vi "Rotator.vi"() -> ()   [LabVIEW 2016]
uses:
  Libraries/Rotator/PerformaxLV_v102.llb/utility_actions.ctl
  Libraries/Rotator/PerformaxLV_v102.llb/commands.ctl
panel:
  in  "stop":bool
  in  "Tab Control":enum32{"Basic controls", "Advanced"}(tab)=enum."Advanced"
  out "In range":bool=TRUE
  out "Status":bool=TRUE
  in  "GO Button":bool
  in  "New position":dbl
  out "Current position":dbl
  in  "Min  angle":dbl=-5.1
  in  "Max angle":dbl=95.1
  in  "Steps per degree":dbl=-780.0
  in  "Redefine Button":bool
  in  "Current position is...":dbl
  out "error out":errorcluster
  out "Status array":bool[](array[boolean])
  out "Status U16":u16
  out "Rotator picture":refnum<vi>(3d-picture)
  # "90"
  # "0"
  # "90"
  # "0"
  # "0"
  # "-90"
  # "0"
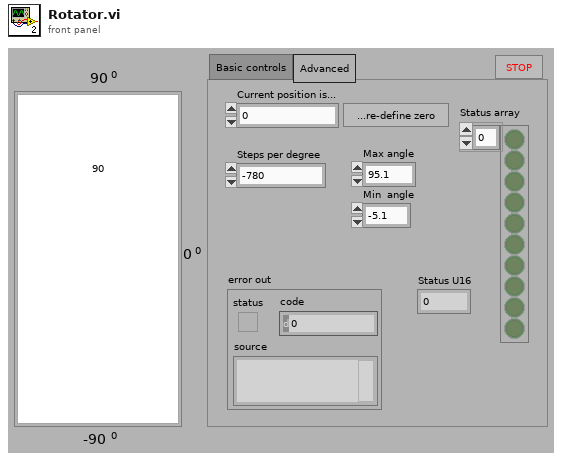
[diagram p1: front panel]
types:
  T1 = typedef "commands.ctl" = enum16{"clearErr", "constJogNeg", "constJogPos", "getAccel", "getDeviceId", "getFirmwareVer", "getHighSpeed", "getIdleAmp", "getLowSpeed", "getMicroStep", "getMotorStatus", "getPolarity", "getPosition", "getProdId", "getPwrStatus", "getRunAmp", "getStatus", "getTemp", "homeNeg", "homePos", "moveToPosition", "powerDown", "powerUp", "setAccel", "setDeviceId", "setHighSpeed", "setIdleAmp", "setLowSpeed", "setMicroStep", "setPolarityLow", "setPolarityHigh", "setPosition", "setRunAmp", "stopFast", "stopSlow"}
  T2 = typedef "utility_actions.ctl" = enum16{"clearError", "closeRef", "demo", "getAcceleration", "getDeviceId", "getDeviceList", "getDriverPowerStatus", "getFirmwareVer", "getHighSpeed", "getIdleCurrent", "getLowSpeed", "getMicroStep", "getMotorStatus", "getPolarity", "getPosition", "getProductId", "getRunCurrent", "getStatus", "getTemperature", "homeMotorNeg", "homeMotorPos", "initialize", "jogConstNeg", "jogConstPos", "moveToPos", "openRef", "pause", "powerOFF", "powerON", "processEvents", "rawCmd", "setAcceleration", "setDeviceId", "setHighSpeed", "setLowSpeed", "setMicroStep", "setPolHigh", "setPolLow", "setPosition", "setRunCurrent", "setIdleCurrent", "setTimeOuts", "stopImmediately", "stopSlowly", "updatePanelItems", "validateDemoPos", "validatePos", "waitUntilDone", "zeroPosition"}
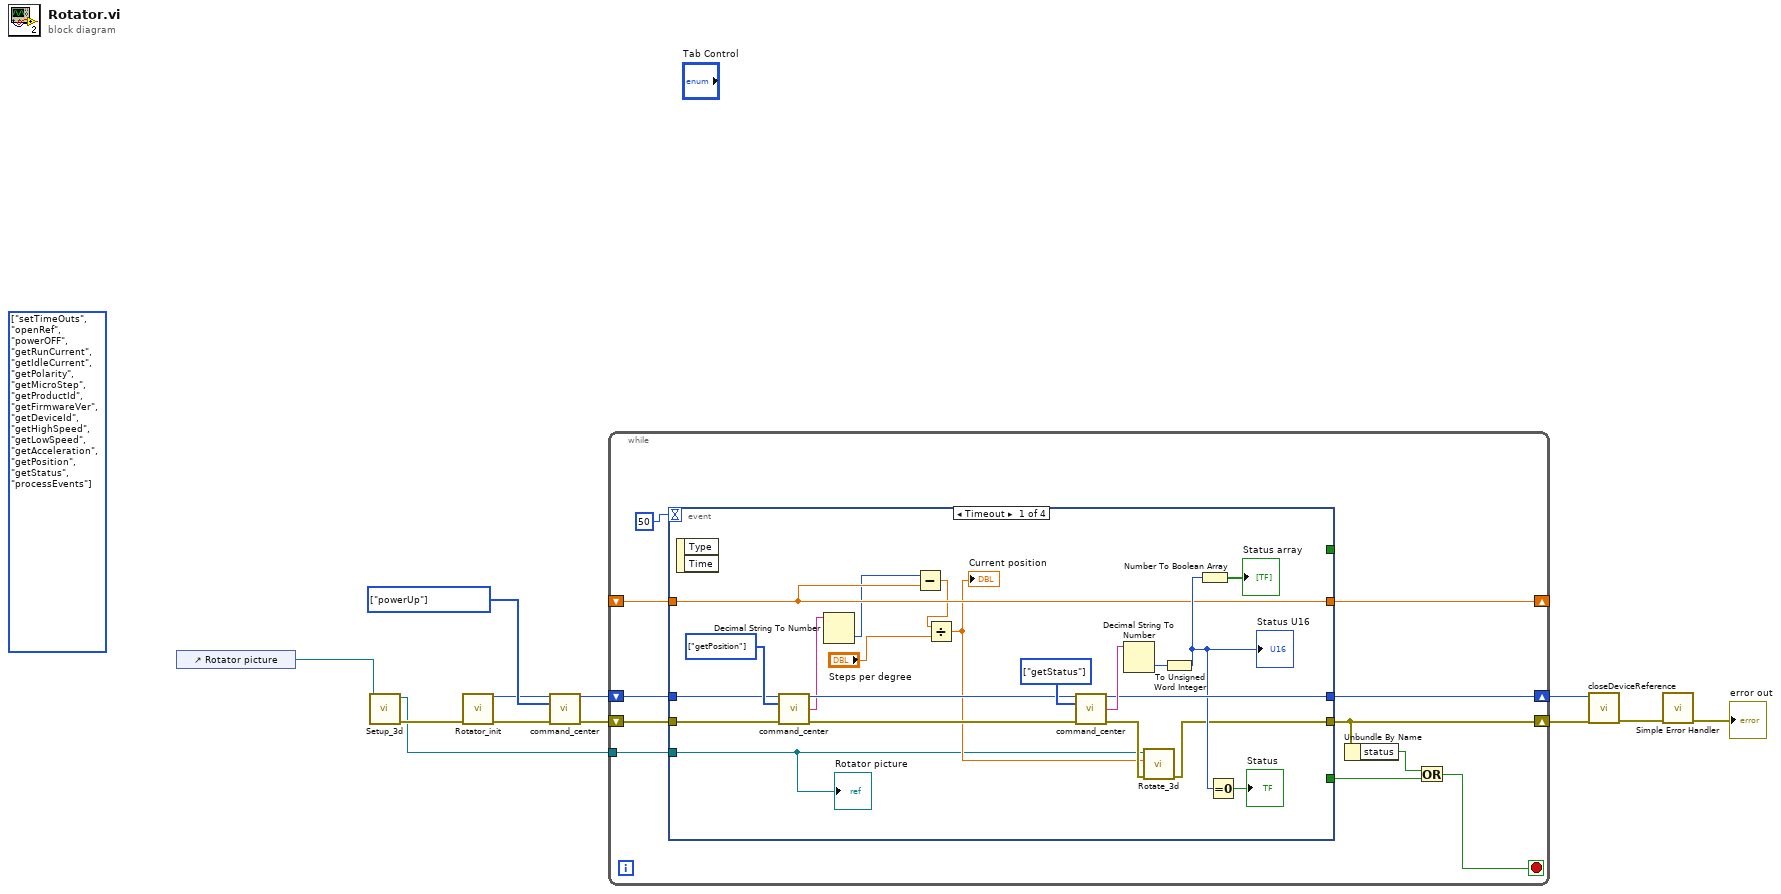
[diagram p0: block diagram]
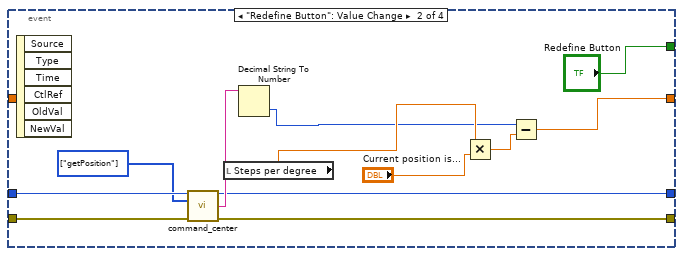
[diagram p2: hidden frame]
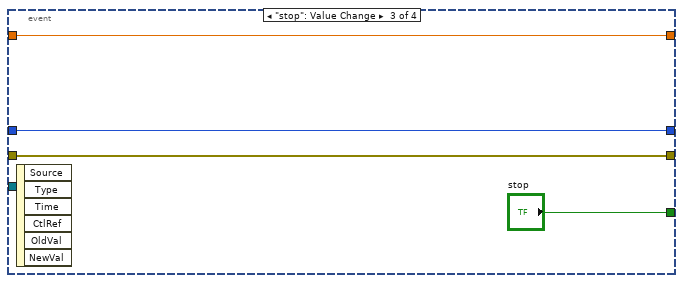
[diagram p3: hidden frame]
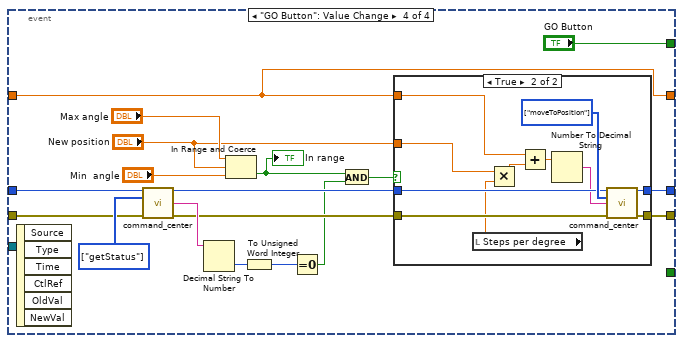
[diagram p4: hidden frame]
diagram:
  w11 = T1[] [enum."powerUp"] items=["clearErr", "constJogNeg", "constJogPos", "getAccel", "getDeviceId", "getFirmwareVer", "getHighSpeed", "getIdleAmp", "getLowSpeed", "getMicroStep", "getMotorStatus", "getPolarity", "getPosition", "getProdId", "getPwrStatus", "getRunAmp", "getStatus", "getTemp", "homeNeg", "homePos", "moveToPosition", "powerDown", "powerUp", "setAccel", "setDeviceId", "setHighSpeed", "setIdleAmp", "setLowSpeed", "setMicroStep", "setPolarityLow", "setPolarityHigh", "setPosition", "setRunAmp", "stopFast", "stopSlow"] ("commands")
  (unwired) T2[] [enum."setTimeOuts", enum."openRef", enum."powerOFF", enum."getRunCurrent", enum."getIdleCurrent", enum."getPolarity", enum."getMicroStep", enum."getProductId", enum."getFirmwareVer", enum."getDeviceId", enum."getHighSpeed", enum."getLowSpeed", enum."getAcceleration", enum."getPosition", enum."getStatus", enum."processEvents"] items=["clearError", "closeRef", "demo", "getAcceleration", "getDeviceId", "getDeviceList", "getDriverPowerStatus", "getFirmwareVer", "getHighSpeed", "getIdleCurrent", "getLowSpeed", "getMicroStep", "getMotorStatus", "getPolarity", "getPosition", "getProductId", "getRunCurrent", "getStatus", "getTemperature", "homeMotorNeg", "homeMotorPos", "initialize", "jogConstNeg", "jogConstPos", "moveToPos", "openRef", "pause", "powerOFF", "powerON", "processEvents", "rawCmd", "setAcceleration", "setDeviceId", "setHighSpeed", "setLowSpeed", "setMicroStep", "setPolHigh", "setPolLow", "setPosition", "setRunCurrent", "setIdleCurrent", "setTimeOuts", "stopImmediately", "stopSlowly", "updatePanelItems", "validateDemoPos", "validatePos", "waitUntilDone", "zeroPosition"] ("actions")
  n1 = control-ref of="Rotator picture"() -> (w3:refnum<vi>)
  n2 = call "Setup_3d.vi"("reference"=w3) -> ("error out"=w2:errorcluster, "Scene reference out"=w1:refnum<vi>)  [unwired: 1 in, 8 out]
  n3 = call "Rotator_init.vi"("error in (no error)"=w2) -> ("error out"=w12:errorcluster, "reference"=w10:i32)  [unwired: 1 in, 8 out]
  n4 = call "command_center.vi"("reference (in)"=w10, "commands"=w11, "error in (no error)"=w12) -> ("reference (out)"=w4:i32, "error out"=w5:errorcluster)  [unwired: 1 in, 10 out]
  n5 = while {
    shift-right: [w18] -> w8
    shift-left: w5 -> [w22]
    shift-right: [w20] -> w7
    shift-left: w4 -> [w21]
    shift-right: [w14] -> _
    shift-left: _ -> [w19]
    tunnel: w1 -> [w13]
    stop <- w15 stop-if-true
    n6 = event shown="[0] Timeout" {
      selector: _ -> [_ _ _ _]
      dyn-events: _ -> [_ _ _ _]
      timeout: 50 -> [_ _ _ _]
      tunnel: [_ _ "stop" _] -> w16
      tunnel: w22 -> [w37 w53 w59 w67]
      tunnel: [w28 w51 w59 w77] -> w18
      tunnel: w21 -> [w36 w54 w58 w65]
      tunnel: [w35 w50 w58 w73] -> w20
      tunnel: w19 -> [w30 _ w57 w72]
      tunnel: [_ "Redefine Button" _ "GO Button"] -> _
      tunnel: [w30 w45 w57 w72] -> w14
      tunnel: w13 -> [w24 _ _ _]
      event Timeout {
        w41 = T1[] [enum."getStatus"] items=["clearErr", "constJogNeg", "constJogPos", "getAccel", "getDeviceId", "getFirmwareVer", "getHighSpeed", "getIdleAmp", "getLowSpeed", "getMicroStep", "getMotorStatus", "getPolarity", "getPosition", "getProdId", "getPwrStatus", "getRunAmp", "getStatus", "getTemp", "homeNeg", "homePos", "moveToPosition", "powerDown", "powerUp", "setAccel", "setDeviceId", "setHighSpeed", "setIdleAmp", "setLowSpeed", "setMicroStep", "setPolarityLow", "setPolarityHigh", "setPosition", "setRunAmp", "stopFast", "stopSlow"] ("commands")
        w38 = T1[] [enum."getPosition"] items=["clearErr", "constJogNeg", "constJogPos", "getAccel", "getDeviceId", "getFirmwareVer", "getHighSpeed", "getIdleAmp", "getLowSpeed", "getMicroStep", "getMotorStatus", "getPolarity", "getPosition", "getProdId", "getPwrStatus", "getRunAmp", "getStatus", "getTemp", "homeNeg", "homePos", "moveToPosition", "powerDown", "powerUp", "setAccel", "setDeviceId", "setHighSpeed", "setIdleAmp", "setLowSpeed", "setMicroStep", "setPolarityLow", "setPolarityHigh", "setPosition", "setRunAmp", "stopFast", "stopSlow"] ("commands")
        n7 = event-data() -> ()  [unwired: 3 out]
        n8 = call "command_center.vi"("reference (in)"=w36, "commands"=w38, "error in (no error)"=w37) -> ("reference (out)"=w40:i32, "data (out)"=w34:string, "error out"=w39:errorcluster)  [unwired: 1 in, 9 out]
        n9 = Decimal String To Number(string=w34) -> (number=w27:i32)  [unwired: 3 out]
        n10 = Subtract(x=w27, y=w30) -> (x-y=w26:dbl)
        n11 = Divide(x=w26, y="Steps per degree") -> (x/y=w25:dbl)
        "Current position" <- w25
        n12 = call "command_center.vi"("reference (in)"=w40, "commands"=w41, "error in (no error)"=w39) -> ("reference (out)"=w35:i32, "data (out)"=w42:string, "error out"=w29:errorcluster)  [unwired: 1 in, 9 out]
        n13 = Decimal String To Number(string=w42) -> (number=w43:i32)  [unwired: 3 out]
        n14 = call "Rotate_3d.vi"("error in (no error)"=w29, "Angle"=w25, "Scene Object"=w24) -> ("error out"=w28:errorcluster)  [unwired: 8 out]
        n15 = To Unsigned Word Integer(number=w43) -> (unsigned 16bit integer=w31:u16)
        "Status U16" <- w31
        n16 = Number To Boolean Array(number=w31) -> (Boolean array=→"Status array":bool[])
        n17 = Equal To 0?(x=w31) -> (x = 0?=→"Status":bool)
        "Rotator picture" <- w24
      }
      event "Redefine Button": Value Change {
        w52 = T1[] [enum."getPosition"] items=["clearErr", "constJogNeg", "constJogPos", "getAccel", "getDeviceId", "getFirmwareVer", "getHighSpeed", "getIdleAmp", "getLowSpeed", "getMicroStep", "getMotorStatus", "getPolarity", "getPosition", "getProdId", "getPwrStatus", "getRunAmp", "getStatus", "getTemp", "homeNeg", "homePos", "moveToPosition", "powerDown", "powerUp", "setAccel", "setDeviceId", "setHighSpeed", "setIdleAmp", "setLowSpeed", "setMicroStep", "setPolarityLow", "setPolarityHigh", "setPosition", "setRunAmp", "stopFast", "stopSlow"] ("commands")
        n18 = event-data() -> ()  [unwired: 7 out]
        n19 = call "command_center.vi"("reference (in)"=w54, "commands"=w52, "error in (no error)"=w53) -> ("reference (out)"=w50:i32, "data (out)"=w55:string, "error out"=w51:errorcluster)  [unwired: 1 in, 9 out]
        n20 = local read "Steps per degree"() -> (w49:dbl)
        n21 = Decimal String To Number(string=w55) -> (number=w46:i32)  [unwired: 3 out]
        n22 = Multiply(x=w49, y="Current position is...") -> (x*y=w47:dbl)
        n23 = Subtract(x=w46, y=w47) -> (x-y=w45:dbl)
      }
      event "stop": Value Change {
        n24 = event-data() -> ()  [unwired: 7 out]
      }
      event "GO Button": Value Change {
        w70 = T1[] [enum."getStatus"] items=["clearErr", "constJogNeg", "constJogPos", "getAccel", "getDeviceId", "getFirmwareVer", "getHighSpeed", "getIdleAmp", "getLowSpeed", "getMicroStep", "getMotorStatus", "getPolarity", "getPosition", "getProdId", "getPwrStatus", "getRunAmp", "getStatus", "getTemp", "homeNeg", "homePos", "moveToPosition", "powerDown", "powerUp", "setAccel", "setDeviceId", "setHighSpeed", "setIdleAmp", "setLowSpeed", "setMicroStep", "setPolarityLow", "setPolarityHigh", "setPosition", "setRunAmp", "stopFast", "stopSlow"] ("commands")
        n25 = event-data() -> ()  [unwired: 7 out]
        n26 = call "command_center.vi"("reference (in)"=w65, "commands"=w70, "error in (no error)"=w67) -> ("reference (out)"=w64:i32, "data (out)"=w69:string, "error out"=w66:errorcluster)  [unwired: 1 in, 9 out]
        n27 = Decimal String To Number(string=w69) -> (number=w68:i32)  [unwired: 3 out]
        n28 = In Range and Coerce(upper limit="Max angle", x="New position", lower limit="Min  angle") -> (In Range?=w61:bool)  [unwired: 1 out]
        "In range" <- w61
        n29 = To Unsigned Word Integer(number=w68) -> (unsigned 16bit integer=w71:u16)
        n30 = Equal To 0?(x=w71) -> (x = 0?=w62:bool)
        n31 = And(x=w61, y=w62) -> (x .and. y?=w63:bool)
        n32 = case shown="True" w63 {
          tunnel: w66 -> [w80 w90]
          tunnel: [w80 w89] -> w77
          tunnel: "New position" -> [_ w84]
          tunnel: w64 -> [w79 w88]
          tunnel: [w79 w87] -> w73
          tunnel: w72 -> [_ w82]
          frame False {
          }
          frame True {
            w91 = T1[] [enum."moveToPosition"] items=["clearErr", "constJogNeg", "constJogPos", "getAccel", "getDeviceId", "getFirmwareVer", "getHighSpeed", "getIdleAmp", "getLowSpeed", "getMicroStep", "getMotorStatus", "getPolarity", "getPosition", "getProdId", "getPwrStatus", "getRunAmp", "getStatus", "getTemp", "homeNeg", "homePos", "moveToPosition", "powerDown", "powerUp", "setAccel", "setDeviceId", "setHighSpeed", "setIdleAmp", "setLowSpeed", "setMicroStep", "setPolarityLow", "setPolarityHigh", "setPosition", "setRunAmp", "stopFast", "stopSlow"] ("commands")
            n33 = local read "Steps per degree"() -> (w86:dbl)
            n34 = Multiply(x=w84, y=w86) -> (x*y=w83:dbl)
            n35 = Add(x=w82, y=w83) -> (x+y=w81:dbl)
            n36 = Number To Decimal String(number=w81) -> (decimal integer string=w85:string)  [unwired: 1 out]
            n37 = call "command_center.vi"("reference (in)"=w88, "commands"=w91, "data (in)"=w85, "error in (no error)"=w90) -> ("reference (out)"=w87:i32, "error out"=w89:errorcluster)  [unwired: 10 out]
          }
        }
      }
    }
    n38 = Unbundle By Name(w18) -> ("status"=w17:bool)
    n39 = Or(x=w17, y=w16) -> (x .or. y?=w15:bool)
  }
  n40 = call "closeDeviceReference.vi"("reference"=w7, "error in (no error)"=w8) -> ("error out"=w9:errorcluster)  [unwired: 1 in, 12 out]
  n41 = call <vilib>:"Simple Error Handler.vi"("error in (no error)"=w9) -> ("error out"=→"error out":errorcluster)  [unwired: 1 in, 7 out]
